vi "Self Msg Send.vi"(9 "Msg EnQ":refnum<class "Msg EnQ.lvclass">, 10 "Msg":refnum<class "Msg.lvclass">, 11 "Self Actor in":refnum<class "Self Actor.lvclass">) -> (0 "error out":errorcluster)   [LabVIEW 2021, in "AAM.lvlib" / "Self Actor.lvclass"]
uses:
  Self Actor.lvclass
  Msg/Msg.lvclass
  Msg EnQ/Msg EnQ.lvclass
  Self Actor.lvclass/Self Actor.ctl
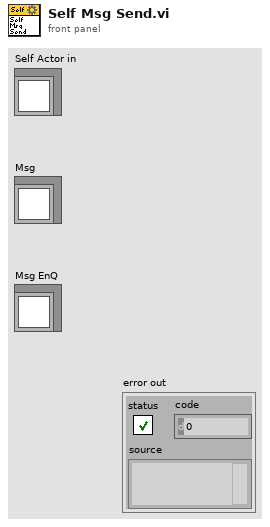
[diagram p1: front panel]
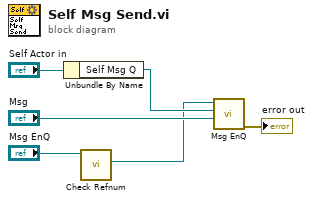
[diagram p0: block diagram]
diagram:
  n1 = Unbundle By Name("Self Actor in") -> ("Self Msg Q"=w4:refnum<class "Msg Q.lvclass">)
  n2 = call "Check Refnum.vi"("Msg EnQ in"="Msg EnQ") -> ("Msg EnQ out"=w1:refnum<class "Msg EnQ.lvclass">)  [unwired: 10 in]
  n3 = call-dynamic "Msg EnQ.vi"("Msg"="Msg", "Msg Q"=w4, "Msg EnQ in"=w1) -> ("error out"=→"error out":errorcluster)  [unwired: 8 in]
